vi "Update resolution.vi"(8 "error in (no error)":errorcluster, 11 "DAQMH121119OrcaFlash in":refnum<class "DAQOrcaFlash.lvclass">) -> (0 "error out":errorcluster, 3 "DAQMH121119OrcaFlash out":refnum<class "DAQOrcaFlash.lvclass">)   [LabVIEW 2012, in "DAQOrcaFlash.lvclass"]
uses:
  DAQOrcaFlash.lvclass
  DAQOrcaFlash.lvclass/DAQOrcaFlash.ctl
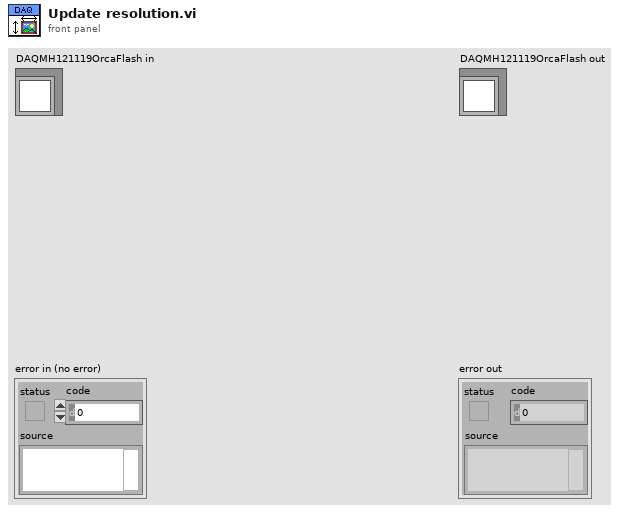
[diagram p1: front panel]
types:
  T1 = cluster{"Horizontal Offset":i32, "Vertical Offset":i32, "Horizontal Width":i32, "Vertical Width":i32}
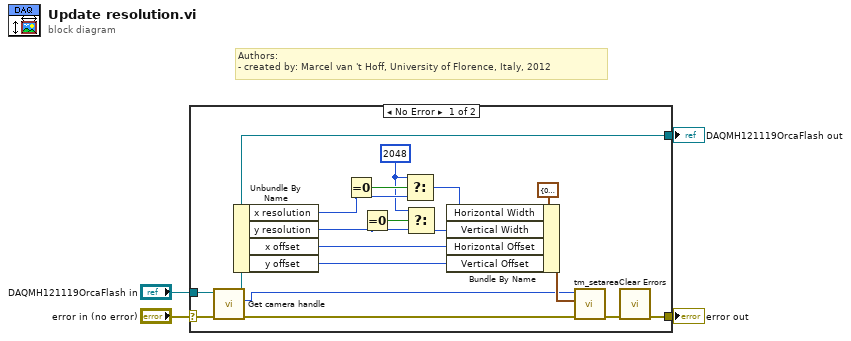
[diagram p0: block diagram]
diagram:
  # "Authors: \n- created by: Marcel van 't Hoff, University of Florence, Italy, 2012"
  n1 = case shown="No Error" "error in (no error)" {
    selector: "error in (no error)" -> [w22 w24]
    tunnel: [w5 w24] -> w3
    tunnel: [w20 w23] -> w1
    tunnel: "DAQMH121119OrcaFlash in" -> [w21 w23]
    frame No Error {
      w7 = 2048 ("t")
      n2 = call "Get camera handle.vi"("error in (no error)"=w22, "DAQMH121119OrcaFlash in"=w21) -> ("error out"=w19:errorcluster, "cam handle"=w14:u32, "DAQMH121119OrcaFlash out"=w20:refnum<class "DAQOrcaFlash.lvclass">)  [unwired: 7 in]
      n3 = Unbundle By Name(w20) -> ("x resolution"=w12:i32, "y resolution"=w10:i32, "x offset"=w17:i32, "y offset"=w16:i32)
      n4 = Equal To 0?(x=w12) -> (x = 0?=w13:bool)
      n5 = Equal To 0?(x=w10) -> (x = 0?=w8:bool)
      n6 = Select(t=w7, s=w13, f=w12) -> (s? t:f=w11:i32)
      n7 = Select(t=w7, s=w8, f=w10) -> (s? t:f=w9:i32)
      n8 = Bundle By Name(cluster=T1 {"Horizontal Offset"=0, "Vertical Offset"=0, "Horizontal Width"=0, "Vertical Width"=0} ("Sub Region"), "Horizontal Width"=w11, "Vertical Width"=w9, "Horizontal Offset"=w17, "Vertical Offset"=w16) -> (w15:T1)
      n9 = call <userlib>:"tm_setarea.vi"("error in (no error)"=w19, "Sub Region"=w15, "Handle in"=w14) -> ("error out"=w6:errorcluster)  [unwired: 7 in, 1 out]
      n10 = call <vilib>:"Clear Errors.vi"("error in (no error)"=w6) -> ("error out"=w5:errorcluster)  [unwired: 6 in]
    }
    frame Error {
    }
  }
  "error out" <- w3
  "DAQMH121119OrcaFlash out" <- w1
